vi "Processing Loop.vi"(8 "error in":errorcluster, 11 "Broker in":refnum<class "Broker.lvclass">) -> (0 "error out":errorcluster, 3 "Broker out":refnum<class "Broker.lvclass">)   [LabVIEW 2014, in "Broker.lvclass"]
uses:
  Broker.lvclass
  Topic_class/Topic.lvclass
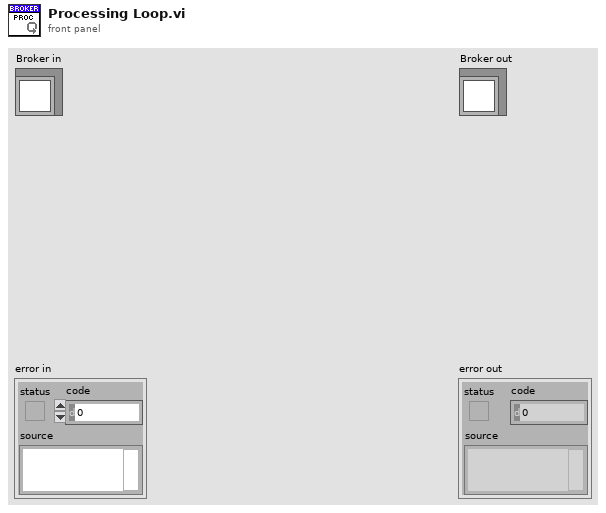
[diagram p1: front panel]
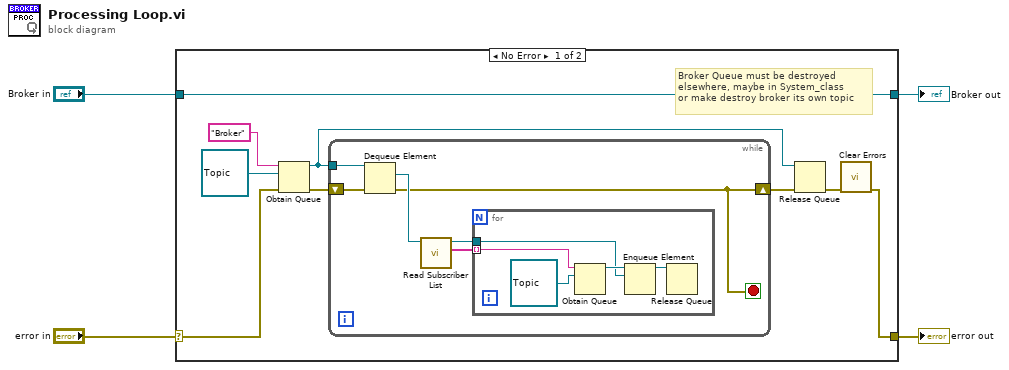
[diagram p0: block diagram]
diagram:
  n1 = case shown="No Error" "error in" {
    selector: "error in" -> [w7 w26]
    tunnel: [w5 w26] -> w3
    tunnel: [w13 w25] -> w1
    tunnel: "Broker in" -> [w13 w25]
    frame No Error {
      # "Broker Queue must be destroyed\nelsewhere, maybe in System_class\nor make destroy broker its own topic"
      n2 = Obtain Queue(name (unnamed)="Broker", element data type=refnum<class "Topic.lvclass"> refnum ("Topic.lvclass"), error in (no error)=w7) -> (queue out=w8:refnum<queue>, error out=w10:errorcluster)  [unwired: 2 in, 1 out]
      n3 = while {
        tunnel: w8 -> [w19]
        shift-right: [w14] -> w9
        shift-left: w10 -> [w18]
        stop <- w14 stop-if-true
        n4 = Dequeue Element(queue=w19, error in (no error)=w18) -> (element=w17:refnum<class "Topic.lvclass">, error out=w14:errorcluster)  [unwired: 1 in, 2 out]
        n5 = call-dynamic "Read Subscriber List.vi"("Topic in"=w17) -> ("Subscriber List"=w16:string[], "Topic out"=w15:refnum<class "Topic.lvclass">)  [unwired: 8 in, 1 out]
        n6 = for {
          tunnel: w16 -> [w21] mode=indexing
          tunnel: w15 -> [w20]
          n7 = Obtain Queue(name (unnamed)=w21, element data type=refnum<class "Topic.lvclass"> refnum ("Topic.lvclass")) -> (queue out=w23:refnum<queue>)  [unwired: 3 in, 2 out]
          n8 = Enqueue Element(queue=w23, element=w20) -> (queue out=w24:refnum<queue>)  [unwired: 2 in, 2 out]
          n9 = Release Queue(queue=w24) -> ()  [unwired: 2 in, 3 out]
        }
      }
      n10 = Release Queue(queue=w8, error in (no error)=w9) -> (error out=w6:errorcluster)  [unwired: 1 in, 2 out]
      n11 = call <vilib>:"Clear Errors.vi"("error in (no error)"=w6) -> ("error out"=w5:errorcluster)  [unwired: 5 in, 1 out]
    }
    frame Error {
    }
  }
  "error out" <- w3
  "Broker out" <- w1
